vi "MHEX_CUIT_CRC_OUT.vi"(10 "width (-)":i16=2, 11 "String":string="E9 01 04 57 53 44 01 44") -> (2 "Numeric":u8, 3 "hex integer string":string)   [LabVIEW 2018]
panel:
  out "substring":string
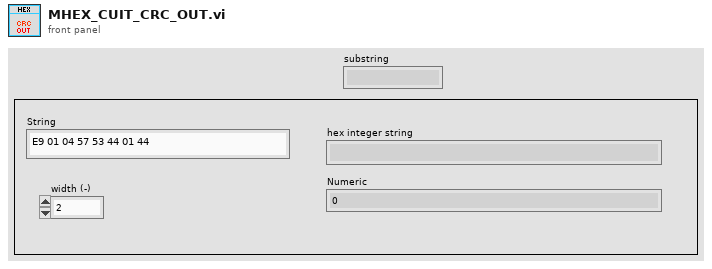
[diagram p1: front panel]
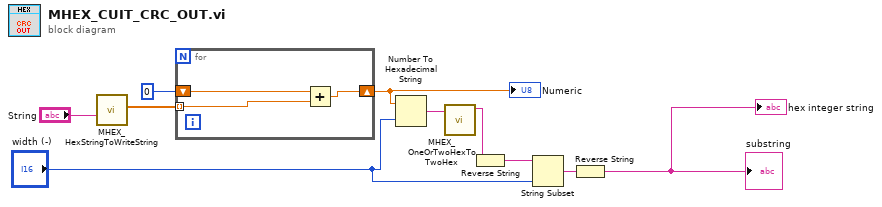
[diagram p0: block diagram]
diagram:
  n1 = call "MHEX_HexStringToWriteString.vi"("STRING HEX"="String") -> ("Hexadecimal array"=w8:dbl[])  [unwired: 7 in, 3 out]
  n2 = for {
    tunnel: w8 -> [w11] mode=indexing
    shift-right: [w12] -> w7
    shift-left: u8 0 -> [w13]
    n3 = Add(x=w13, y=w11) -> (x+y=w12:dbl)
  }
  "Numeric" <- w7
  n4 = Number To Hexadecimal String(1:"width (-)", 2:w7) -> (0:w6:string)
  n5 = call "MHEX_OneOrTwoHexToTwoHex.vi"("HEX In"=w6) -> ("HEX Out"=w4:string)  [unwired: 10 in]
  n6 = Reverse String(1:w4) -> (0:w3:string)
  n7 = String Subset(string=w3, length (rest)="width (-)") -> (substring=w2:string)  [unwired: 1 in]
  n8 = Reverse String(1:w2) -> (0:→"hex integer string" →"substring":string)
